vi "NXT_MIDBRAIN_BEHAVIOR Forebrain Control.vi"(2 "Behavior #":i32, 3 "_behaviorWeights":T2=[0, 0, 0, 0, 0, 0], 4 "_fromPC":u8[](array[numeric])=[0, 0, 0, 0, 0, 0, 0, 0, 0, 0, 0]) -> (0 "_behaviorOutput":T1, 1 "_FBirTheta":i8)   [LabVIEW 2012]
uses:
  behaviorWeights_t.ctl
  behaviorOutput_t.ctl
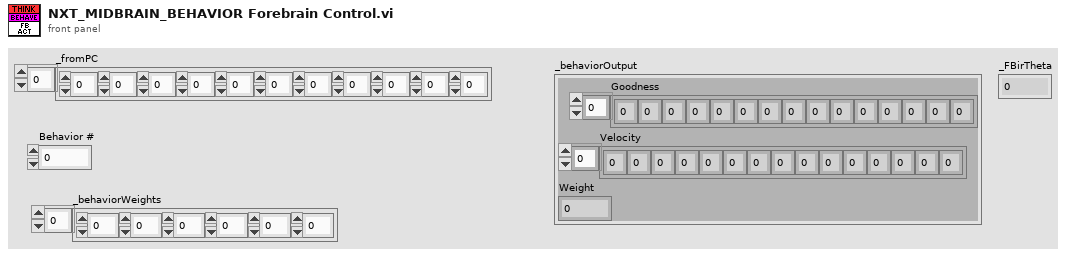
[diagram p1: front panel]
types:
  T1 = typedef "behaviorOutput_t.ctl" = cluster{"Goodness":i8[], "Velocity":i8[], "Weight":i8}
  T2 = typedef "behaviorWeights_t.ctl" = i8[]
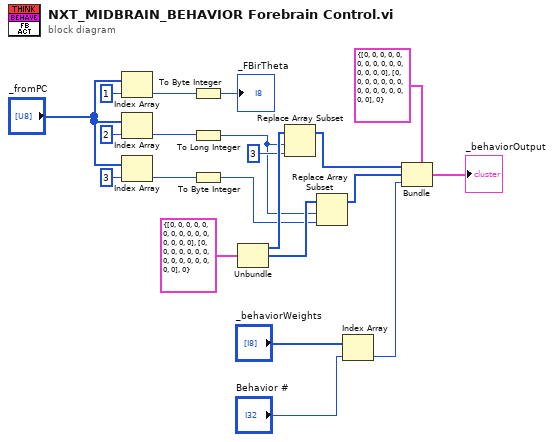
[diagram p0: block diagram]
diagram:
  n1 = Index Array(array="_fromPC", index=1) -> (element=w4:u8)
  n2 = Index Array(array="_fromPC", index=2) -> (element=w3:u8)
  n3 = Index Array(array="_fromPC", index=3) -> (element=w2:u8)
  n4 = To Byte Integer(number=w4) -> (8bit integer=→"_FBirTheta":i8)
  n5 = To Long Integer(number=w3) -> (32bit integer=w13:i32)
  n6 = To Byte Integer(number=w2) -> (8bit integer=w12:i8)
  n7 = Unbundle(T1 {"Goodness"=[0, 0, 0, 0, 0, 0, 0, 0, 0, 0, 0, 0, 0, 0, 0], "Velocity"=[0, 0, 0, 0, 0, 0, 0, 0, 0, 0, 0, 0, 0, 0, 0], "Weight"=0} ("Behavior Output")) -> ("Goodness"=w18:i8[], "Velocity"=w15:i8[])  [unwired: 1 out]
  n8 = Replace Array Subset(array=w18, new element=i8 3 ("new element/subarray"), index=w13) -> (w17:i8[])
  n9 = Replace Array Subset(array=w15, new element=w12, index=w13) -> (w14:i8[])
  n10 = Index Array(array="_behaviorWeights", index="Behavior #") -> (element=w9:i8)
  n11 = Bundle(cluster=T1 {"Goodness"=[0, 0, 0, 0, 0, 0, 0, 0, 0, 0, 0, 0, 0, 0, 0], "Velocity"=[0, 0, 0, 0, 0, 0, 0, 0, 0, 0, 0, 0, 0, 0, 0], "Weight"=0} ("Behavior Output"), "Goodness"=w17, "Velocity"=w14, "Weight"=w9) -> (→"_behaviorOutput":T1)
